vi "GPIB_364Xa.vi"(1 "level (0.0 volts)":dbl caption="SET VOLT" format="%.2p", 2 "limit (0.0)":dbl caption="I LIMIT" format="%.2p", 4 "limit (22.0 volts)":dbl=22.0 caption="OVP LIMIT" format="%.2p", 5 "Output Enabled":bool, 6 "error in (no error)":errorcluster {"code" format="%.0x"}, 7 "Enum":T1(ring)=enum."Output Control", 8 "Instrument Select (Output 1)":string(combo)="OUT1", 9 "VISA resource name":refnum<visa-resource-name>) -> (0 "error out":errorcluster, 3 "Result":dbl)   [LabVIEW 2014]
doc: "This VI controls an Agilent GPIB Dual Power supply. The routines are:\n\nInit (initialze handle)\nSetup (set OVP, OCP, Set Voltage)\nRead Volatge\nRead Current\nOutput Control"
panel:
  out "VISA resource name out":refnum<visa-resource-name>
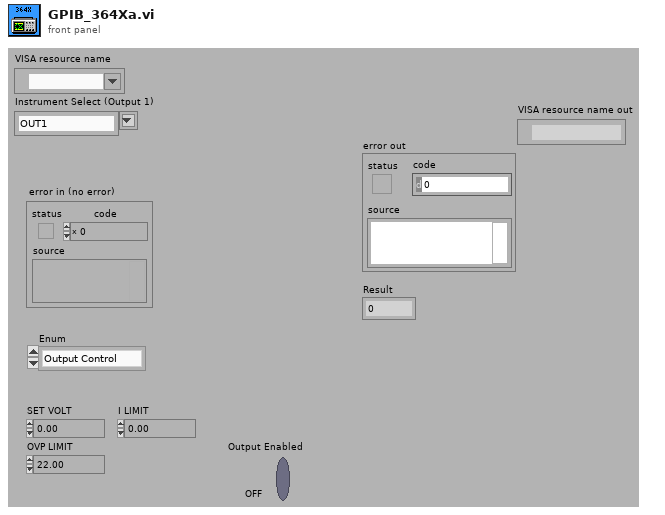
[diagram p1: front panel]
types:
  T1 = enum16{"Idle", "Init", "Setup", "Output Control", "Read Voltage", "Read Current", "DeInit Power Supply"}
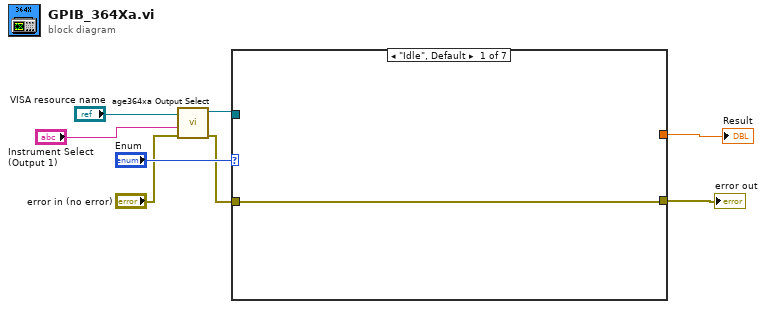
[diagram p0: block diagram]
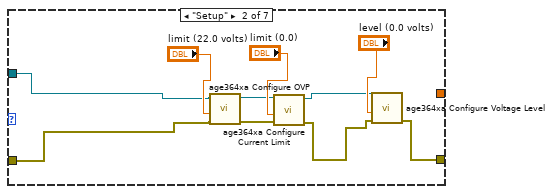
[diagram p2: hidden frame]
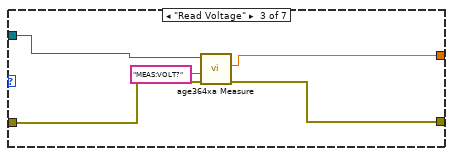
[diagram p3: hidden frame]
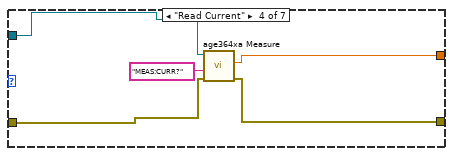
[diagram p4: hidden frame]
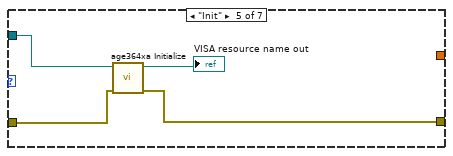
[diagram p5: hidden frame]
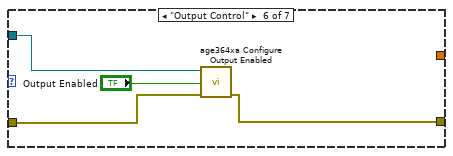
[diagram p6: hidden frame]
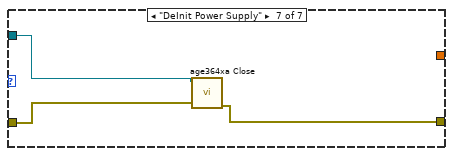
[diagram p7: hidden frame]
diagram:
  n1 = call "age364xa Output Select.vi"("error in (no error)"="error in (no error)", "Instrument Select (Output 1)"="Instrument Select (Output 1)", "VISA session"="VISA resource name") -> ("error out"=w2:errorcluster, "dup VISA session"=w1:refnum<visa-resource-name>)  [unwired: 7 in]
  n2 = case shown="\"Idle\", Default" "Enum" {
    tunnel: w2 -> [w9 w19 w24 w28 w33 w35 w39]
    tunnel: [w9 w15 w21 w27 w32 w36 w40] -> w7
    tunnel: [_ _ w23 w26 _ _ _] -> w6
    tunnel: w1 -> [_ w10 w20 w25 w31 w34 w38]
    frame "Idle", Default {
    }
    frame "Setup" {
      n3 = call "age364xa Configure OVP.vi"("error in (no error)"=w19, "Limit (22.0 Volts)"="limit (22.0 volts)", "VISA session"=w10) -> ("error out"=w11:errorcluster, "dup VISA session"=w12:refnum<visa-resource-name>)  [unwired: 7 in]
      n4 = call "age364xa Configure Current Limit.vi"("error in (no error)"=w11, "Current Limit (0.0 Amps)"="limit (0.0)", "VISA session"=w12) -> ("error out"=w16:errorcluster, "dup VISA session"=w17:refnum<visa-resource-name>)  [unwired: 7 in]
      n5 = call "age364xa Configure Voltage Level.vi"("error in (no error)"=w16, "Level (0.0 Volts)"="level (0.0 volts)", "VISA session"=w17) -> ("error out"=w15:errorcluster)  [unwired: 7 in, 1 out]
    }
    frame "Read Voltage" {
      n6 = call "age364xa Measure.vi"("error in (no error)"=w24, "Measurement Type (Voltage)"="MEAS:VOLT?", "VISA session"=w20) -> ("error out"=w21:errorcluster, "Measurement"=w23:dbl)  [unwired: 6 in, 1 out]
    }
    frame "Read Current" {
      n7 = call "age364xa Measure.vi"("error in (no error)"=w28, "Measurement Type (Voltage)"="MEAS:CURR?", "VISA session"=w25) -> ("error out"=w27:errorcluster, "Measurement"=w26:dbl)  [unwired: 6 in, 1 out]
    }
    frame "Init" {
      n8 = call "age364xa Initialize.vi"("error in (no error)"=w33, "Instrument Resource Name"=w31) -> ("error out"=w32:errorcluster, "dup VISA session"=→"VISA resource name out":refnum<visa-resource-name>)  [unwired: 8 in]
    }
    frame "Output Control" {
      n9 = call "age364xa Configure Output Enabled.vi"("error in (no error)"=w35, "Output Enabled (F: Off)"="Output Enabled", "VISA session"=w34) -> ("error out"=w36:errorcluster)  [unwired: 7 in, 1 out]
    }
    frame "DeInit Power Supply" {
      n10 = call "age364xa Close.vi"("error in (no error)"=w39, "VISA session"=w38) -> ("error out"=w40:errorcluster)  [unwired: 9 in]
    }
  }
  "error out" <- w7
  "Result" <- w6
